vi "Done Button_TEST.vi"() -> ()   [LabVIEW 2023]
uses:
  Done Button.ctl
panel:
  in  "Done 2":T1
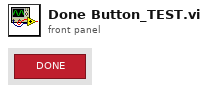
[diagram p1: front panel]
types:
  T1 = typedef "Done Button.ctl" = bool
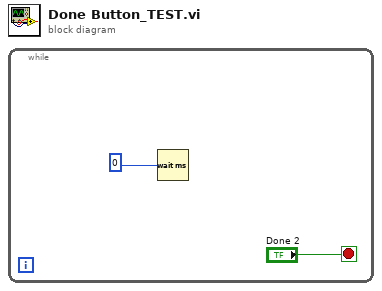
[diagram p0: block diagram]
diagram:
  n1 = while {
    stop <- "Done 2" stop-if-true
    n2 = Wait (ms)(milliseconds to wait=u32 0) -> ()  [unwired: 1 out]
  }
